vi "TimeBelowThreshold.vi"(3 "Current Value":dbl=20.0, 4 "Threshold":dbl=20.0) -> (1 "Time Below":u32)   [LabVIEW 2018]
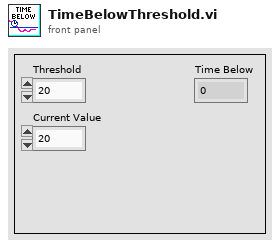
[diagram p1: front panel]
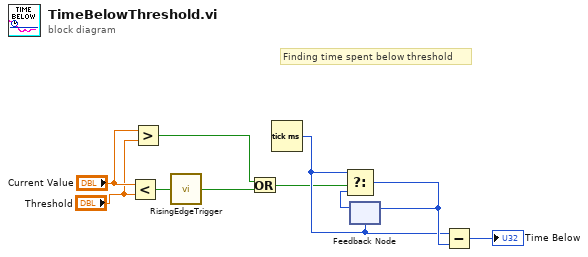
[diagram p0: block diagram]
diagram:
  # "Finding time spent below threshold"
  n1 = Less?(x="Current Value", y="Threshold") -> (x < y?=w10:bool)
  n2 = Greater?(x="Current Value", y="Threshold") -> (0:w1:bool)
  n3 = call "RisingEdgeTrigger.vi"("Raw Signal"=w10) -> ("Trigger"=w9:bool)
  n4 = Or(x=w1, y=w9) -> (x .or. y?=w4:bool)
  n5 = Tick Count (ms)() -> (millisecond timer value=w6:u32)
  n6 = feedback #1(w6) -> (w8:u32)
  n7 = Select(t=w6, s=w4, f=w8) -> (s? t:f=w7:u32)
  n8 = feedback-in #1(w7) -> ()
  n9 = Subtract(x=w6, y=w7) -> (x-y=→"Time Below":u32)
